vi "ATM_Server.vi"() -> ()   [LabVIEW 2020]
uses:
  <vilib>/Utility/file.llb/Read Delimited Spreadsheet (string).vi
  <vilib>/Utility/file.llb/Write Delimited Spreadsheet (string).vi
  <vilib>/regexp/Match Regular Expression.xnode
panel:
  out "concatenated string":string
  out "x = y?":bool
  out "data out":string
  out "Operation Error Out":errorcluster
  out "Login Error Out":errorcluster
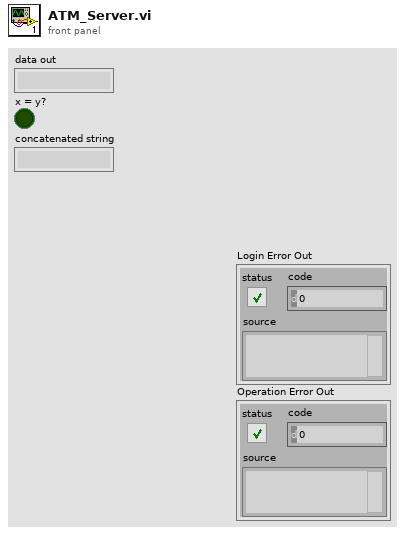
[diagram p1: front panel]
types:
  T1 = enum16{"Welcome", "Start machine", "Sign in machine"}
  T2 = enum16{"open", "replace", "create", "open or create", "replace or create", "replace or create with confirmation"}
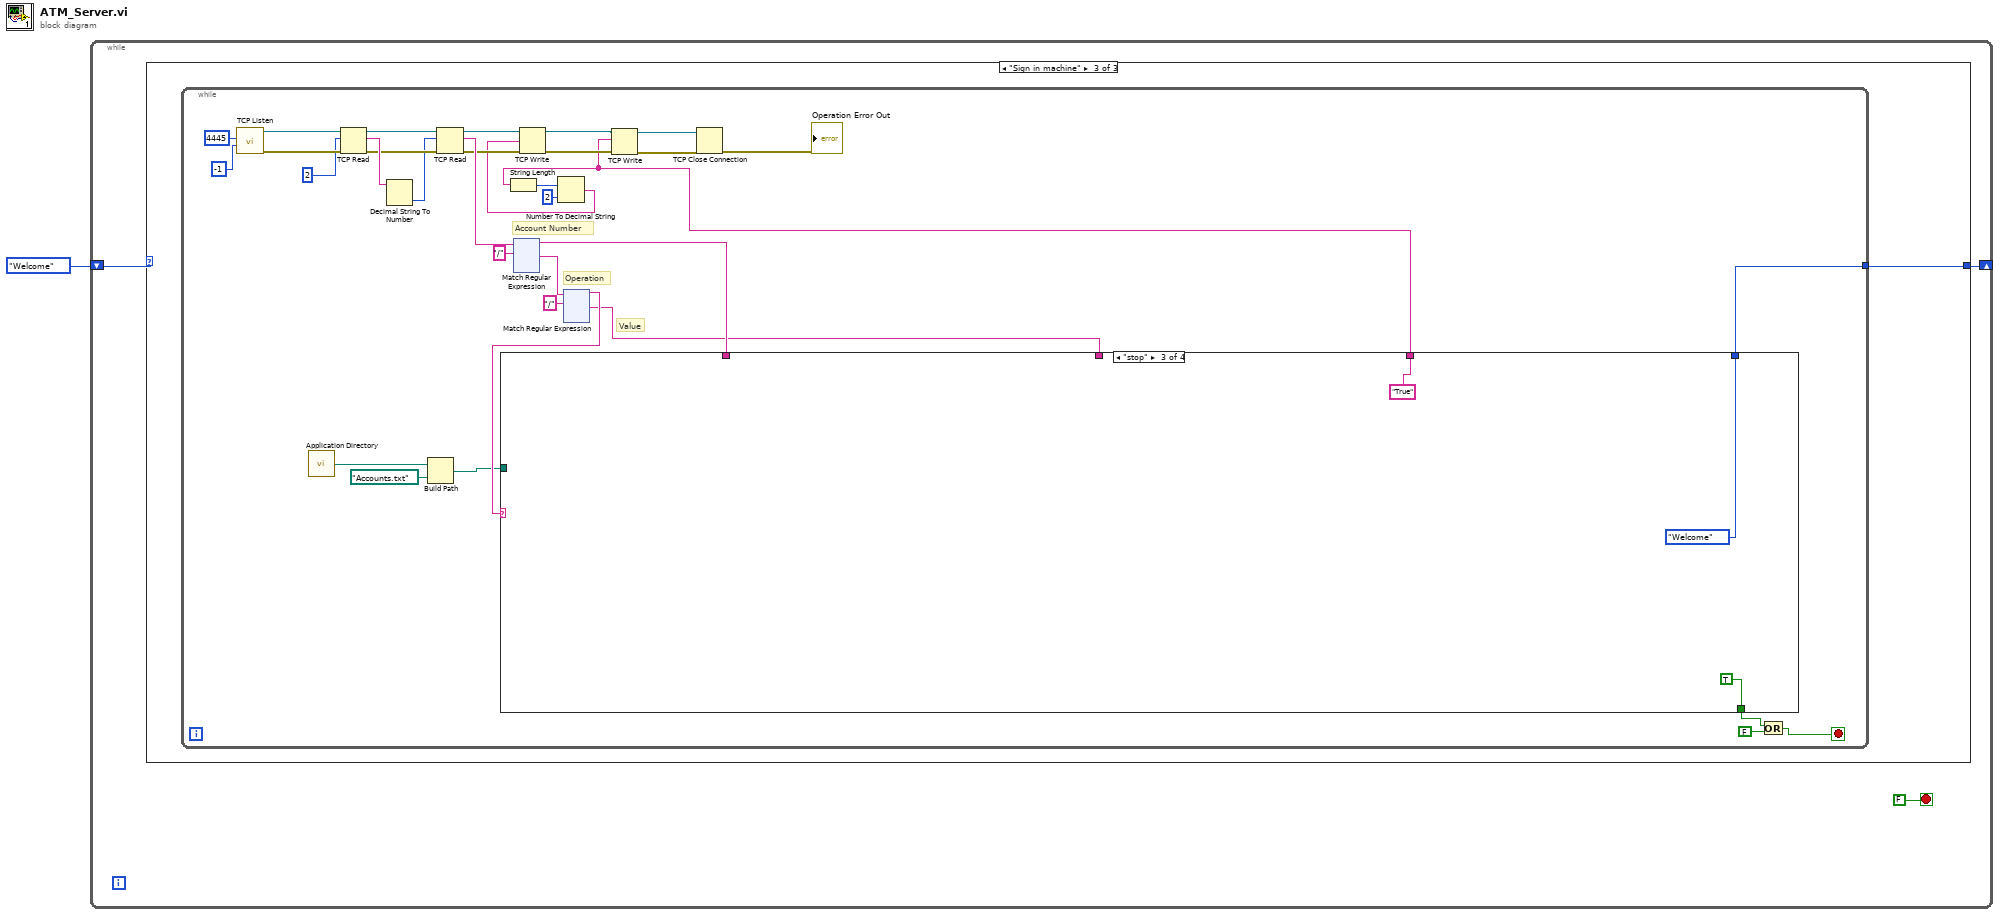
[diagram p0: block diagram]
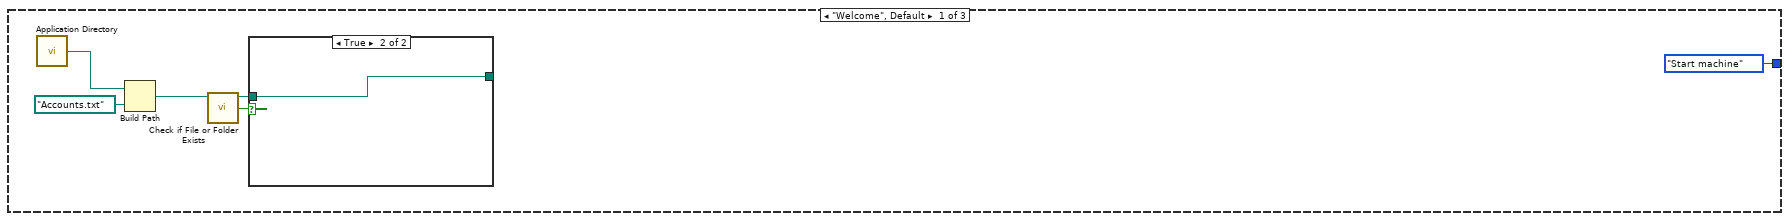
[diagram p2: hidden frame]
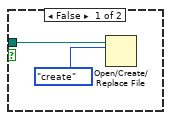
[diagram p3: hidden frame]
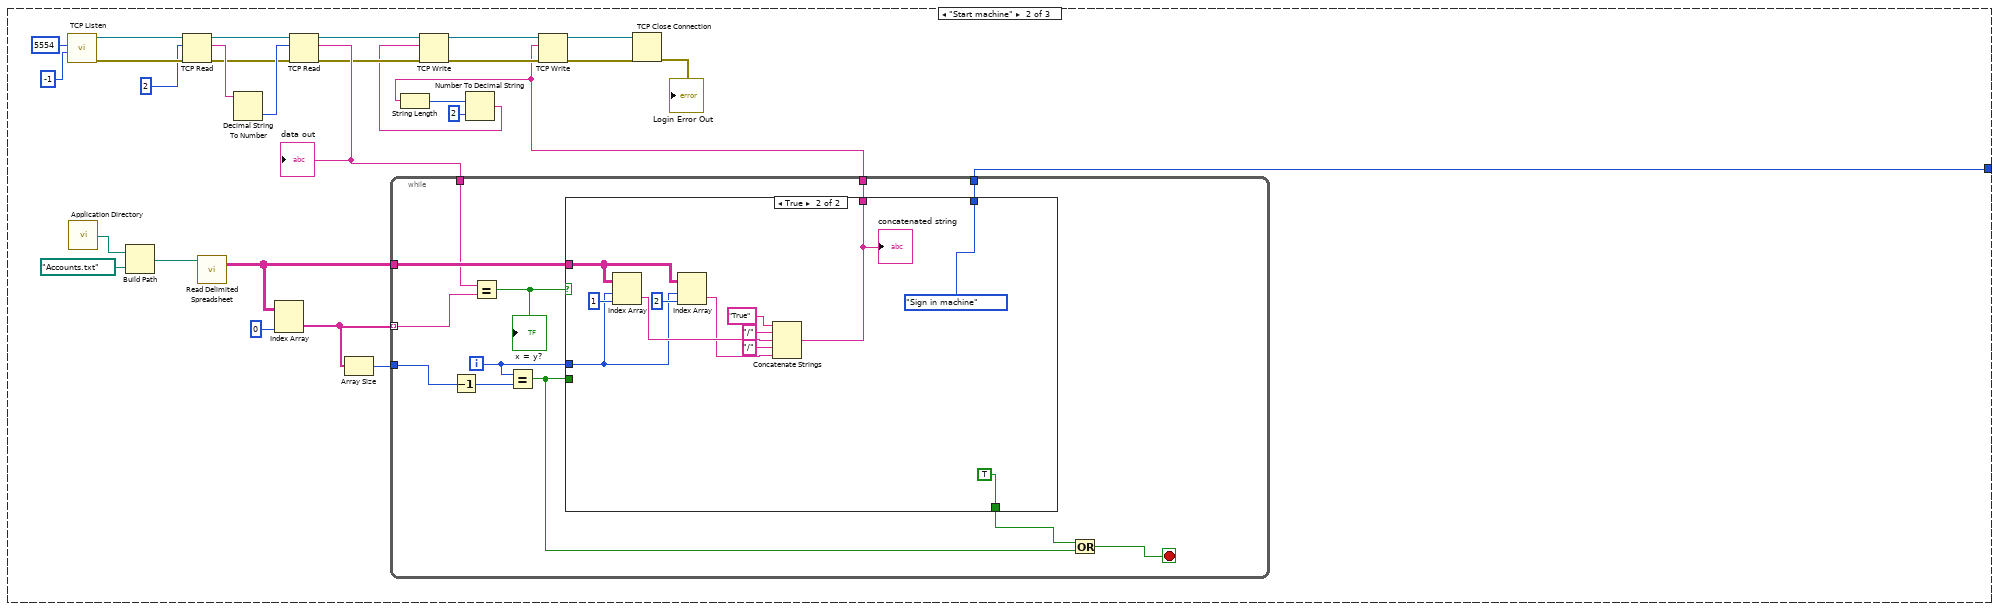
[diagram p4: hidden frame]
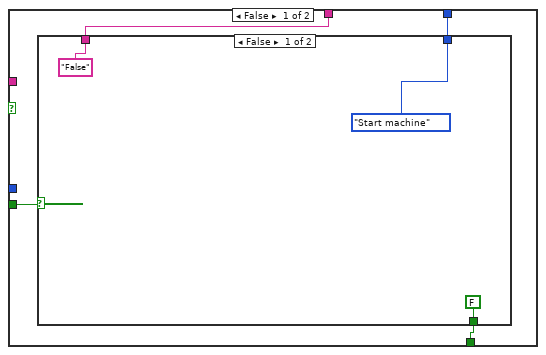
[diagram p5: hidden frame]
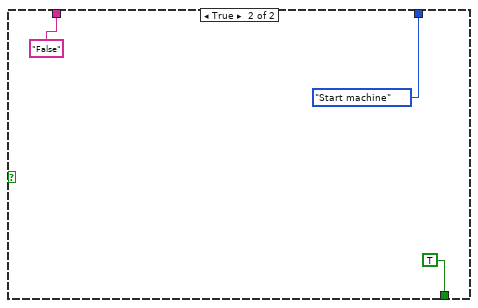
[diagram p6: hidden frame]
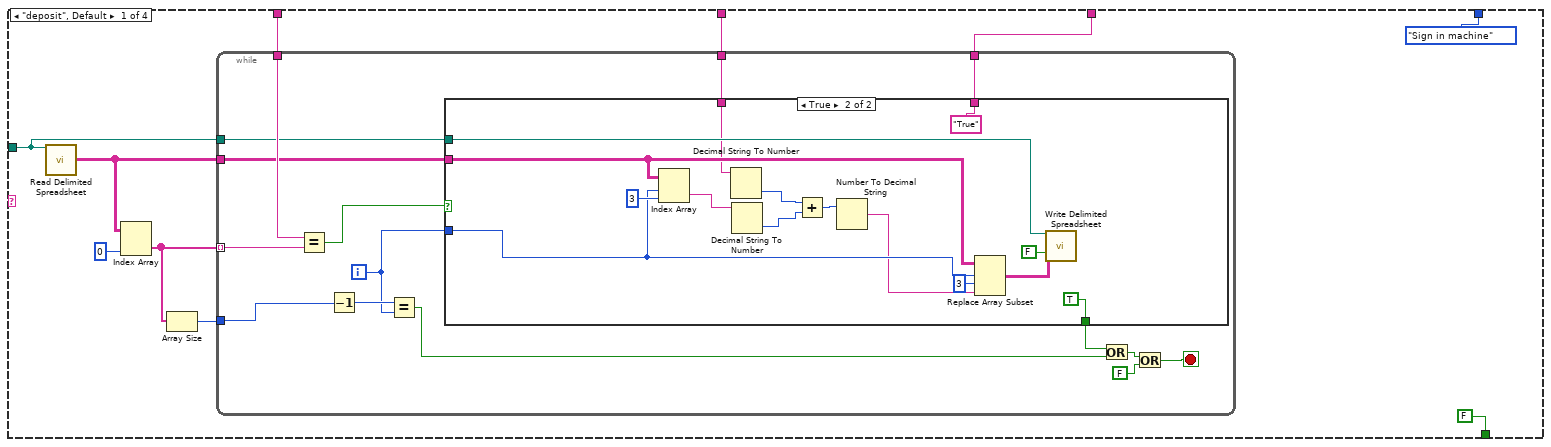
[diagram p7: hidden frame]
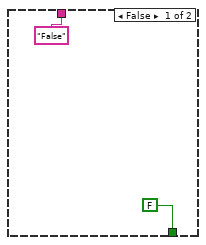
[diagram p8: hidden frame]
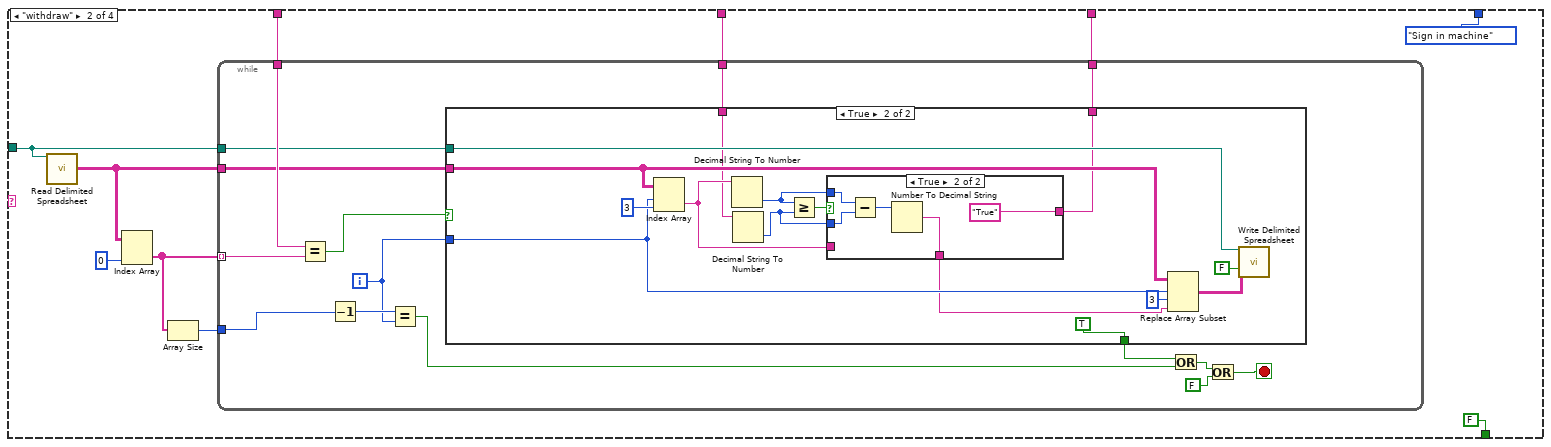
[diagram p9: hidden frame]
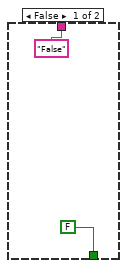
[diagram p10: hidden frame]
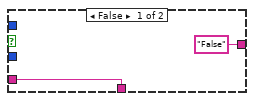
[diagram p11: hidden frame]
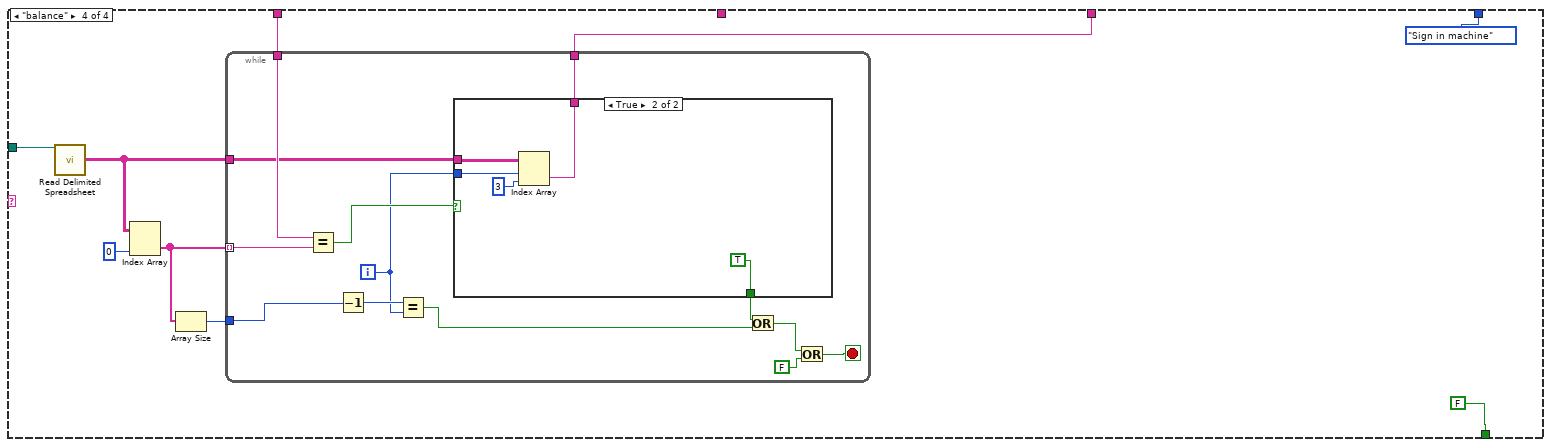
[diagram p12: hidden frame]
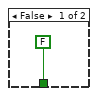
[diagram p13: hidden frame]
diagram:
  n1 = while {
    shift-right: [w2] -> _
    shift-left: T1."Welcome" ("Enum") -> [w3]
    stop <- FALSE stop-if-true
    n2 = case shown="\"Sign in machine\"" w3 {
      tunnel: [T1."Start machine" ("Enum") w14 w77] -> w2
      frame "Welcome", Default {
        n3 = call <vilib>:"Application Directory.vi"() -> ("Application Directory"=w7:path)
        n4 = Build Path(base path=w7, name or relative path=path "Accounts.txt") -> (appended path=w8:path)
        n5 = call <vilib>:"Check if File or Folder Exists.vi"("path"=w8) -> ("file or folder exists?"=w9:bool, "dup path"=w10:path)  [unwired: 8 in, 1 out]
        n6 = case shown="True" w9 {
          tunnel: w10 -> [w11 w13]
          tunnel: [_ w13] -> _
          frame False {
            n7 = Open/Create/Replace File(file path (use dialog)=w11, operation (0:open)=T2."create") -> ()  [unwired: 4 in, 3 out]
          }
          frame True {
          }
        }
      }
      frame "Start machine" {
        n8 = call <vilib>:"TCP Listen.vi"("timeout ms (wait forever: -1)"=-1, "port"=u16 5554) -> ("error out"=w33:errorcluster, "connection ID"=w32:refnum<k5>)  [unwired: 5 in, 3 out]
        n9 = call <vilib>:"Application Directory.vi"() -> ("Application Directory"=w37:path)
        n10 = Build Path(base path=w37, name or relative path=path "Accounts.txt") -> (appended path=w38:path)
        n11 = TCP Read(connection ID=w32, bytes to read=2, error in (no error)=w33) -> (connection ID out=w31:refnum<k5>, data out=w35:string, error out=w34:errorcluster)  [unwired: 2 in]
        n12 = call-poly <vilib>:"Read Delimited Spreadsheet.vi"("file path (dialog if empty)"=w38) -> ("all rows"=w39:string[][])  [unwired: 9 in, 5 out]
        n13 = Decimal String To Number(string=w35) -> (number=w36:i32)  [unwired: 2 in, 1 out]
        n14 = Index Array "Index Array"(array=w39, index (col)=0 ("disabled index (col)")) -> (element=w40:string[])  [unwired: 1 in]
        n15 = TCP Read(connection ID=w31, bytes to read=w36, error in (no error)=w34) -> (connection ID out=w22:refnum<k5>, data out=w42:string, error out=w20:errorcluster)  [unwired: 2 in]
        "data out" <- w42
        n16 = Array Size(array=w40) -> (size(s)=w41:i32)
        n17 = while {
          tunnel: w39 -> [w52]
          tunnel: w40 -> [w49] mode=indexing
          tunnel: w41 -> [w54]
          tunnel: w42 -> [w51]
          tunnel: [w47] -> w16
          tunnel: [w44] -> w14
          i -> [w45]
          stop <- w48 stop-if-true
          n18 = Decrement(x=w54) -> (x-1=w53:i32)
          n19 = Equal?(x=w51, y=w49) -> (x = y?=w50:bool)
          "x = y?" <- w50
          n20 = Equal?(x=w45, y=w53) -> (x = y?=w46:bool)
          n21 = case shown="True" w50 {
            tunnel: w52 -> [_ w73]
            tunnel: [w57 w71] -> w47
            tunnel: w46 -> [w58 _]
            tunnel: [w55 TRUE ("y")] -> w43
            tunnel: w45 -> [_ w67]
            tunnel: [w56 T1."Sign in machine" ("Enum")] -> w44
            frame False {
              n22 = case shown="False" w58 {
                tunnel: ["False" "False"] -> w57
                tunnel: [T1."Start machine" ("Enum") T1."Start machine" ("Enum")] -> w56
                tunnel: [FALSE ("y") TRUE ("y")] -> w55
                frame False {
                }
                frame True {
                }
              }
            }
            frame True {
              n23 = Index Array "Index Array"(array=w73, index (row)=w67, index (col)=1 ("disabled index (col)")) -> (element=w72:string)
              n24 = Index Array(array=w73, index (row)=w67, index (col)=2 ("disabled index (col)")) -> (element=w68:string)
              n25 = Concatenate Strings("True" ("string"), "/" ("string"), w72, "/" ("string"), w68) -> (w71:string)
              "concatenated string" <- w71
            }
          }
          n26 = Or(x=w43, y=w46) -> (x .or. y?=w48:bool)
        }
        n27 = String Length(string=w16) -> (length=w18:i32)
        n28 = Number To Decimal String(number=w18, width (-)=i16 2) -> (decimal integer string=w15:string)
        n29 = TCP Write(connection ID=w22, data in=w15, error in (no error)=w20) -> (connection ID out=w21:refnum<k5>, error out=w19:errorcluster)  [unwired: 1 in, 1 out]
        n30 = TCP Write(connection ID=w21, data in=w16, error in (no error)=w19) -> (connection ID out=w29:refnum<k5>, error out=w28:errorcluster)  [unwired: 1 in, 1 out]
        n31 = TCP Close Connection(connection ID=w29, error in (no error)=w28) -> (error out=→"Login Error Out":errorcluster)  [unwired: 1 in, 1 out]
      }
      frame "Sign in machine" {
        n32 = while {
          tunnel: [w78] -> w77
          stop <- w81 stop-if-true
          # "Value"
          # "Operation"
          # "Account Number"
          n33 = call <vilib>:"TCP Listen.vi"("timeout ms (wait forever: -1)"=-1, "port"=u16 4445) -> ("error out"=w109:errorcluster, "connection ID"=w108:refnum<k5>)  [unwired: 5 in, 3 out]
          n34 = call <vilib>:"Application Directory.vi"() -> ("Application Directory"=w96:path)
          n35 = TCP Read(connection ID=w108, bytes to read=2, error in (no error)=w109) -> (connection ID out=w107:refnum<k5>, data out=w111:string, error out=w110:errorcluster)  [unwired: 2 in]
          n36 = Decimal String To Number(string=w111) -> (number=w84:i32)  [unwired: 2 in, 1 out]
          n37 = Build Path(base path=w96, name or relative path=path "Accounts.txt") -> (appended path=w94:path)
          n38 = TCP Read(connection ID=w107, bytes to read=w84, error in (no error)=w110) -> (connection ID out=w91:refnum<k5>, data out=w100:string, error out=w89:errorcluster)  [unwired: 2 in]
          n39 = xnode ("Match Regular Expression")("input string"=w100, "regular expression"="/") -> ("before match"=w93:string, "after match"=w98:string)  [unwired: 4 in, 3 out]
          n40 = xnode ("Match Regular Expression")("input string"=w98, "regular expression"="/") -> ("before match"=w97:string, "after match"=w92:string)  [unwired: 4 in, 3 out]
          n41 = case shown="\"stop\"" w97 {
            tunnel: w94 -> [w116 w159 _ w214]
            tunnel: w93 -> [w117 w156 _ w210]
            tunnel: [w115 w157 "True" ("String") w208] -> w83
            tunnel: w92 -> [w114 w158 _ _]
            tunnel: [FALSE FALSE TRUE ("y") FALSE] -> w79
            tunnel: [T1."Sign in machine" ("Enum") T1."Sign in machine" ("Enum") T1."Welcome" ("Enum") T1."Sign in machine" ("Enum")] -> w78
            frame "deposit", Default {
              n42 = call-poly <vilib>:"Read Delimited Spreadsheet.vi"("file path (dialog if empty)"=w116) -> ("all rows"=w120:string[][])  [unwired: 9 in, 5 out]
              n43 = Index Array "Index Array"(array=w120, index (col)=0 ("disabled index (col)")) -> (element=w119:string[])  [unwired: 1 in]
              n44 = Array Size(array=w119) -> (size(s)=w118:i32)
              n45 = while {
                tunnel: w120 -> [w131]
                tunnel: w119 -> [w128] mode=indexing
                tunnel: w117 -> [w133]
                tunnel: w118 -> [w130]
                tunnel: w116 -> [w127]
                tunnel: [w126] -> w115
                tunnel: w114 -> [w125]
                i -> [w129]
                stop <- w134 stop-if-true
                n46 = Equal?(x=w133, y=w128) -> (x = y?=w132:bool)
                n47 = Decrement(x=w130) -> (x-1=w135:i32)
                n48 = Equal?(x=w135, y=w129) -> (x = y?=w123:bool)
                n49 = case shown="True" w132 {
                  tunnel: w131 -> [_ w150]
                  tunnel: w129 -> [_ w146]
                  tunnel: w127 -> [_ w153]
                  tunnel: ["False" "True"] -> w126
                  tunnel: w125 -> [_ w147]
                  tunnel: [FALSE TRUE] -> w122
                  frame False {
                  }
                  frame True {
                    n50 = Index Array(array=w150, index (row)=w146, index (col)=3 ("disabled index (col)")) -> (element=w148:string)
                    n51 = Decimal String To Number(string=w147) -> (number=w145:i32)  [unwired: 2 in, 1 out]
                    n52 = Decimal String To Number(string=w148) -> (number=w144:i32)  [unwired: 2 in, 1 out]
                    n53 = Add(x=w145, y=w144) -> (x+y=w143:i32)
                    n54 = Number To Decimal String(number=w143) -> (decimal integer string=w140:string)  [unwired: 1 in]
                    n55 = Replace Array Subset(array=w150, new element=w140, index (row)=w146, index (col)=3 ("disabled index (col)")) -> (w152:string[][])
                    n56 = call-poly <vilib>:"Write Delimited Spreadsheet.vi"("file path (dialog if empty)"=w153, "2D data"=w152, "append to file? (new file:F)"=FALSE) -> ()  [unwired: 11 in, 2 out]
                  }
                }
                n57 = Or(x=w122, y=w123) -> (x .or. y?=w124:bool)
                n58 = Or(x=w124, y=FALSE) -> (x .or. y?=w134:bool)
              }
            }
            frame "withdraw" {
              n59 = call-poly <vilib>:"Read Delimited Spreadsheet.vi"("file path (dialog if empty)"=w159) -> ("all rows"=w161:string[][])  [unwired: 9 in, 5 out]
              n60 = Index Array "Index Array"(array=w161, index (col)=0 ("disabled index (col)")) -> (element=w162:string[])  [unwired: 1 in]
              n61 = Array Size(array=w162) -> (size(s)=w163:i32)
              n62 = while {
                tunnel: w161 -> [w173]
                tunnel: w162 -> [w170] mode=indexing
                tunnel: w156 -> [w175]
                tunnel: w163 -> [w172]
                tunnel: w159 -> [w169]
                tunnel: [w168] -> w157
                tunnel: w158 -> [w167]
                i -> [w171]
                stop <- w176 stop-if-true
                n63 = Equal?(x=w175, y=w170) -> (x = y?=w174:bool)
                n64 = Decrement(x=w172) -> (x-1=w177:i32)
                n65 = Equal?(x=w177, y=w171) -> (x = y?=w165:bool)
                n66 = case shown="True" w174 {
                  tunnel: w173 -> [_ w192]
                  tunnel: w171 -> [_ w183]
                  tunnel: w169 -> [_ w195]
                  tunnel: ["False" w190] -> w168
                  tunnel: w167 -> [_ w184]
                  tunnel: [FALSE TRUE] -> w164
                  frame False {
                  }
                  frame True {
                    n67 = Index Array(array=w192, index (row)=w183, index (col)=3 ("disabled index (col)")) -> (element=w185:string)
                    n68 = Decimal String To Number(string=w185) -> (number=w188:i32)  [unwired: 2 in, 1 out]
                    n69 = Decimal String To Number(string=w184) -> (number=w187:i32)  [unwired: 2 in, 1 out]
                    n70 = Greater Or Equal?(x=w188, y=w187) -> (x >= y?=w189:bool)
                    n71 = case shown="True" w189 {
                      tunnel: ["False" "True"] -> w190
                      tunnel: w188 -> [_ w202]
                      tunnel: w187 -> [_ w201]
                      tunnel: [w196 w199] -> w181
                      tunnel: w185 -> [w196 _]
                      frame False {
                      }
                      frame True {
                        n72 = Subtract(x=w202, y=w201) -> (x-y=w200:i32)
                        n73 = Number To Decimal String(number=w200) -> (decimal integer string=w199:string)  [unwired: 1 in]
                      }
                    }
                    n74 = Replace Array Subset(array=w192, new element=w181, index (row)=w183, index (col)=3 ("disabled index (col)")) -> (w194:string[][])
                    n75 = call-poly <vilib>:"Write Delimited Spreadsheet.vi"("file path (dialog if empty)"=w195, "2D data"=w194, "append to file? (new file:F)"=FALSE) -> ()  [unwired: 11 in, 2 out]
                  }
                }
                n76 = Or(x=w164, y=w165) -> (x .or. y?=w166:bool)
                n77 = Or(x=w166, y=FALSE) -> (x .or. y?=w176:bool)
              }
            }
            frame "stop" {
            }
            frame "balance" {
              n78 = call-poly <vilib>:"Read Delimited Spreadsheet.vi"("file path (dialog if empty)"=w214) -> ("all rows"=w212:string[][])  [unwired: 9 in, 5 out]
              n79 = Index Array "Index Array"(array=w212, index (col)=0 ("disabled index (col)")) -> (element=w211:string[])  [unwired: 1 in]
              n80 = Array Size(array=w211) -> (size(s)=w209:i32)
              n81 = while {
                tunnel: w212 -> [w221]
                tunnel: w211 -> [w224] mode=indexing
                tunnel: w210 -> [w223]
                tunnel: w209 -> [w220]
                tunnel: [w218] -> w208
                i -> [w219]
                stop <- w225 stop-if-true
                n82 = Equal?(x=w223, y=w224) -> (x = y?=w222:bool)
                n83 = Decrement(x=w220) -> (x-1=w226:i32)
                n84 = Equal?(x=w226, y=w219) -> (x = y?=w216:bool)
                n85 = case shown="True" w222 {
                  tunnel: w221 -> [_ w232]
                  tunnel: w219 -> [_ w231]
                  tunnel: [_ w230] -> w218
                  tunnel: [FALSE TRUE] -> w215
                  frame False {
                  }
                  frame True {
                    n86 = Index Array "Index Array"(array=w232, index (row)=w231, index (col)=3 ("disabled index (col)")) -> (element=w230:string)
                  }
                }
                n87 = Or(x=w215, y=w216) -> (x .or. y?=w217:bool)
                n88 = Or(x=w217, y=FALSE) -> (x .or. y?=w225:bool)
              }
            }
          }
          n89 = String Length(string=w83) -> (length=w87:i32)
          n90 = Number To Decimal String(number=w87, width (-)=i16 2) -> (decimal integer string=w85:string)
          n91 = TCP Write(connection ID=w91, data in=w85, error in (no error)=w89) -> (connection ID out=w90:refnum<k5>, error out=w88:errorcluster)  [unwired: 1 in, 1 out]
          n92 = TCP Write(connection ID=w90, data in=w83, error in (no error)=w88) -> (connection ID out=w106:refnum<k5>, error out=w105:errorcluster)  [unwired: 1 in, 1 out]
          n93 = TCP Close Connection(connection ID=w106, error in (no error)=w105) -> (error out=→"Operation Error Out":errorcluster)  [unwired: 1 in, 1 out]
          n94 = Or(x=w79, y=FALSE) -> (x .or. y?=w81:bool)
        }
      }
    }
  }
